vi "Day 24-With Map.vi"() -> ()   [LabVIEW 2021]
uses:
  Day 24-Operation Enum.ctl
  Day 24-Variable Enum.ctl
  <vilib>/Utility/file.llb/Read Delimited Spreadsheet (string).vi
panel:
  out "Array 2":T3(array[cluster])
  out "Model Number":u64
  out "Array":T4(array[cluster])
  in  "Input File":enum32{"example input", "input"}(radio)
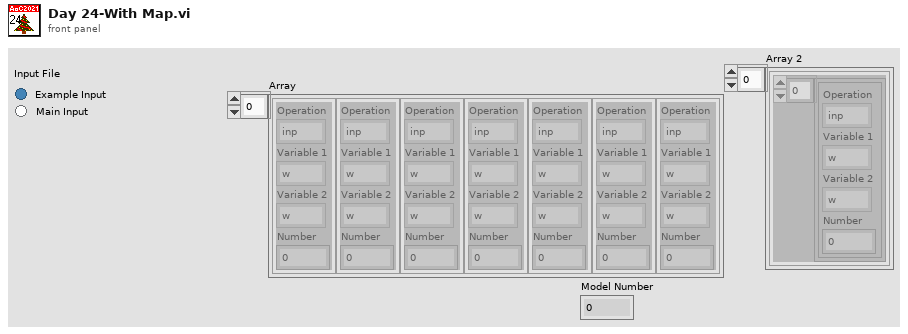
[diagram p1: front panel]
types:
  T1 = typedef "Day 24-Operation Enum.ctl" = enum16{"inp", "add", "mul", "div", "mod", "eql"}
  T2 = typedef "Day 24-Variable Enum.ctl" = enum16{"w", "x", "y", "z", "num"}
  T3 = cluster{cluster{"Operation":T1, "Variable 1":T2, "Variable 2":T2, "Number":i64}[]}[]
  T4 = cluster{"Operation":T1, "Variable 1":T2, "Variable 2":T2, "Number":i64}[]
  T5 = cluster{"Operation":T1, "Variable 1":T2, "Variable 2":T2, "Number":i64}
  T6 = cluster{cluster{"Operation":T1, "Variable 1":T2, "Variable 2":T2, "Number":i64}[]}
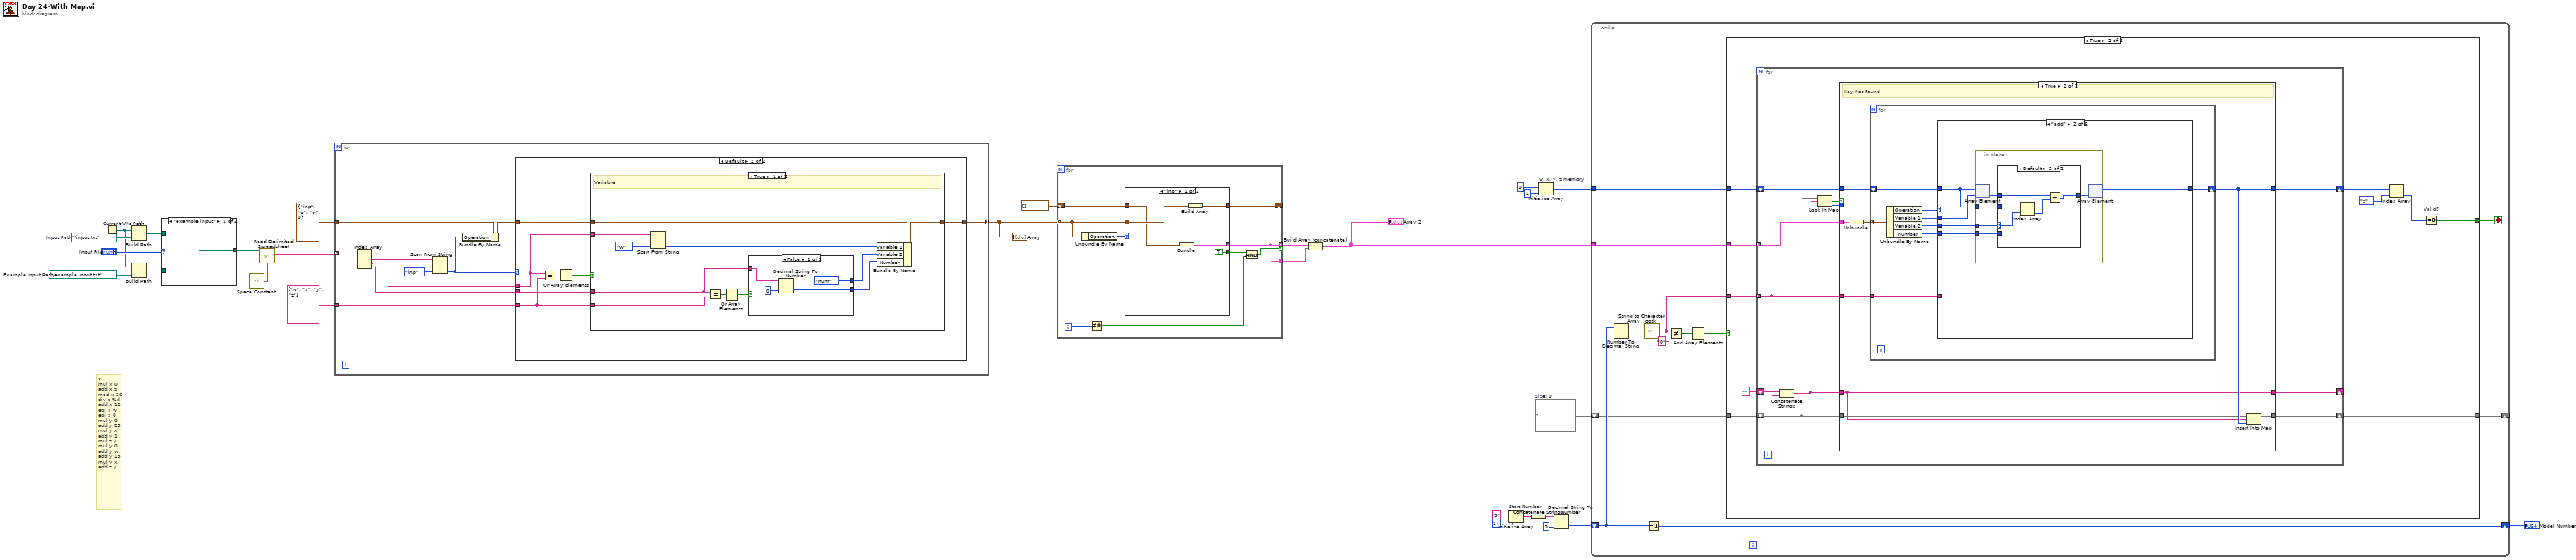
[diagram p0: block diagram]
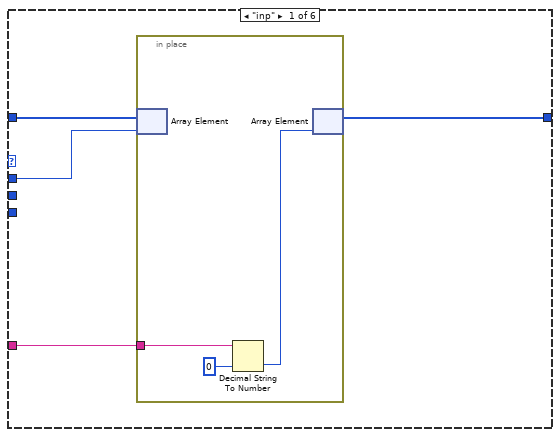
[diagram p4: hidden frame]
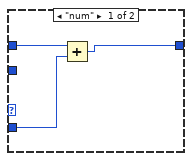
[diagram p5: hidden frame]
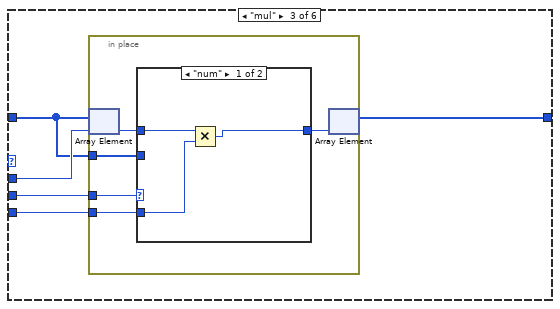
[diagram p6: hidden frame]
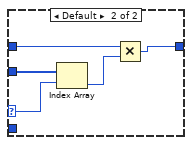
[diagram p7: hidden frame]
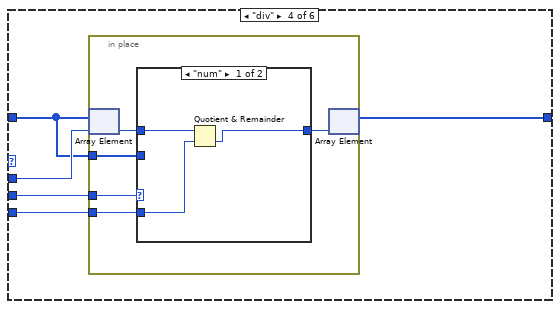
[diagram p8: hidden frame]
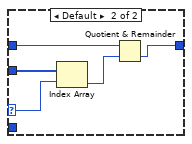
[diagram p9: hidden frame]
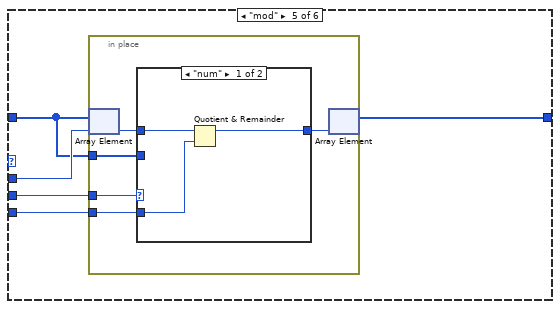
[diagram p10: hidden frame]
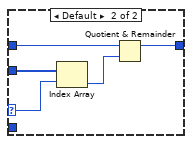
[diagram p11: hidden frame]
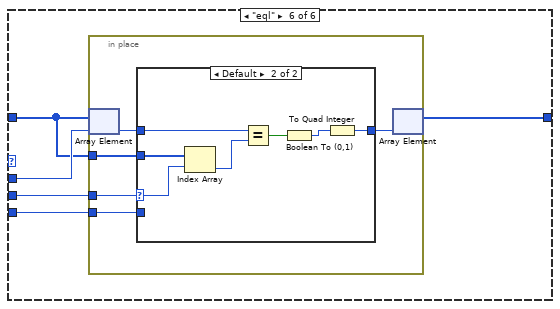
[diagram p12: hidden frame]
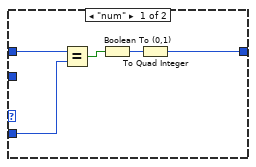
[diagram p13: hidden frame]
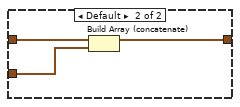
[diagram p14: hidden frame]
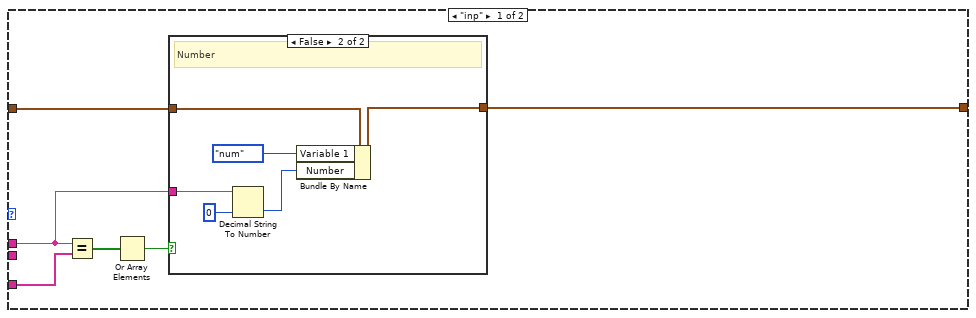
[diagram p15: hidden frame]
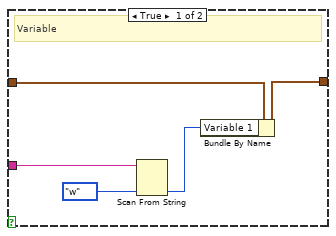
[diagram p16: hidden frame]
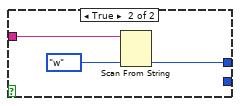
[diagram p17: hidden frame]
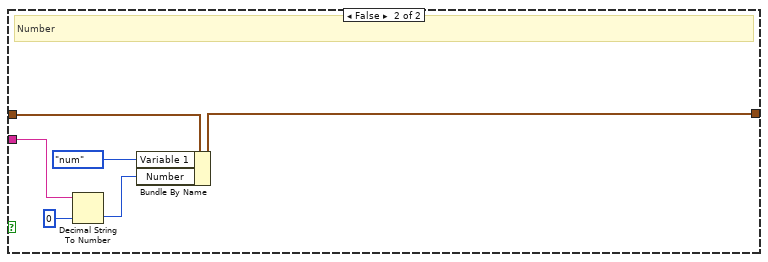
[diagram p18: hidden frame]
diagram:
  w4 = map{string, i64[]} {}  # Size: 0
  w26 = path "../example input.txt"  # Example Input Path
  w27 = path "../input.txt"  # Input Path
  # "w\nmul x 0\nadd x z\nmod x 26\ndiv z %d\nadd x 12\neql x w\neql x 0\nmul y 0\nadd y 25\nmul y x\nadd y 1\nmul z y\nmul y 0\nadd y w\nadd y 15\nmul y x\nadd z y"
  n1 = Current VI's Path() -> (path=w22:path)
  n2 = Build Path(base path=w22, name or relative path=w27) -> (appended path=w24:path)
  n3 = Build Path(base path=w22, name or relative path=w26) -> (appended path=w23:path)
  n4 = case shown="\"example input\"" "Input File" {
    tunnel: w24 -> [_ w29]
    tunnel: w23 -> [w28 _]
    tunnel: [w28 w29] -> w1
    frame "example input" {
    }
    frame "input" {
    }
  }
  n5 = call <vilib>:"Space Constant.vi"() -> ("String"=w19:string)
  n6 = call-poly <vilib>:"Read Delimited Spreadsheet.vi"("file path (dialog if empty)"=w1, "delimiter (\\t)"=w19) -> ("all rows"=w18:string[][])  [unwired: 8 in, 5 out]
  n7 = for {
    tunnel: w18 -> [w34] mode=indexing
    tunnel: string[] ["w", "x", "y", "z"] -> [w39]
    tunnel: T5 {"Operation"=enum."inp", "Variable 1"=enum."w", "Variable 2"=enum."w", "Number"=0} -> [w37]
    tunnel: [w35] -> w17 mode=indexing
    n8 = Index Array(array=w34) -> (element #1=w33:string, element #2=w31:string, element #3=w30:string)  [unwired: 3 in]
    n9 = Scan From String(input string=w33, default 1=Day_24-Operation_Enum."inp") -> (output 1=w36:T1)  [unwired: 3 in, 3 out]
    n10 = Bundle By Name(cluster=w37, "Operation"=w36) -> (w38:T5)
    n11 = case shown="Default" w36 {
      tunnel: w39 -> [w45 w59]
      tunnel: w38 -> [w42 w61]
      tunnel: [w41 w60] -> w35
      tunnel: w31 -> [w40 w58]
      tunnel: w30 -> [_ w57]
      frame "inp" {
        n12 = Equal?(x=w40, y=w45) -> (x = y?=w44:bool[])
        n13 = Or Array Elements(Boolean array=w44) -> (logical OR=w43:bool)
        n14 = case shown="False" w43 {
          tunnel: w42 -> [w50 w56]
          tunnel: w40 -> [w49 w54]
          tunnel: [w46 w55] -> w41
          frame True {
            # "Variable"
            n15 = Scan From String(input string=w49, default 1=Day_24-Variable_Enum."w" ("Variable 1")) -> (output 1=w47:T2)  [unwired: 3 in, 3 out]
            n16 = Bundle By Name(cluster=w50, "Variable 1"=w47) -> (w46:T5)
          }
          frame False {
            # "Number"
            n17 = Decimal String To Number(string=w54, default (0L)=i64 0 ("default (0 I32)")) -> (number=w52:i64)  [unwired: 1 in, 1 out]
            n18 = Bundle By Name(cluster=w56, "Variable 1"=Day_24-Variable_Enum."num", "Number"=w52) -> (w55:T5)
          }
        }
      }
      frame Default {
        n19 = Equal?(x=w58, y=w59) -> (x = y?=w63:bool[])
        n20 = Or Array Elements(Boolean array=w63) -> (logical OR=w62:bool)
        n21 = case shown="True" w62 {
          tunnel: w61 -> [w74 w87]
          tunnel: w58 -> [w73 w85]
          tunnel: [w70 w86] -> w60
          tunnel: w59 -> [w68 _]
          tunnel: w57 -> [w64 _]
          frame True {
            # "Variable"
            n22 = Scan From String(input string=w73, default 1=Day_24-Variable_Enum."w" ("Variable 1")) -> (output 1=w71:T2)  [unwired: 3 in, 3 out]
            n23 = Equal?(x=w64, y=w68) -> (x = y?=w69:bool[])
            n24 = Or Array Elements(Boolean array=w69) -> (logical OR=w67:bool)
            n25 = case shown="False" w67 {
              tunnel: w64 -> [w78 w80]
              tunnel: [Day_24-Variable_Enum."num" ("Variable 1") w79] -> w66
              tunnel: [w77 _] -> w65
              frame False {
                n26 = Decimal String To Number(string=w78, default (0L)=i64 0 ("default (0 I32)")) -> (number=w77:i64)  [unwired: 1 in, 1 out]
              }
              frame True {
                n27 = Scan From String(input string=w80, default 1=Day_24-Variable_Enum."w" ("Variable 1")) -> (output 1=w79:T2)  [unwired: 3 in, 3 out]
              }
            }
            n28 = Bundle By Name(cluster=w74, "Variable 1"=w71, "Variable 2"=w66, "Number"=w65) -> (w70:T5)
          }
          frame False {
            # "Number"
            n29 = Decimal String To Number(string=w85, default (0L)=i64 0 ("default (0 I32)")) -> (number=w83:i64)  [unwired: 1 in, 1 out]
            n30 = Bundle By Name(cluster=w87, "Variable 1"=Day_24-Variable_Enum."num", "Number"=w83) -> (w86:T5)
          }
        }
      }
    }
  }
  "Array" <- w17
  n31 = for {
    tunnel: w17 -> [w95] mode=indexing
    shift-right: [w94] -> _
    shift-left: T4 [] -> [w93]
    tunnel: [w88] -> w5 mode=indexing if=w91
    tunnel: [w88] -> w2
    i -> [w90]
    n32 = Unbundle By Name(w95) -> ("Operation"=w96:T1)
    n33 = Not Equal To 0?(x=w90) -> (x != 0?=w89:bool)
    n34 = case shown="\"inp\"" w96 {
      tunnel: w95 -> [w101 w104]
      tunnel: [w100 w103] -> w94
      tunnel: w93 -> [w98 w102]
      tunnel: [w99 _] -> w88
      tunnel: [TRUE _] -> w92
      frame "inp" {
        n35 = Bundle(w98) -> (w99:T6)  [unwired: 1 in]
        n36 = Build Array(w101) -> (w100:T4)
      }
      frame Default {
        n37 = Build Array (concatenate)(w102, w104) -> (w103:T4)
      }
    }
    n38 = And(x=w92, y=w89) -> (x .and. y?=w91:bool)
  }
  n39 = Build Array (concatenate)(w5, w2) -> (w3:T3)
  "Array 2" <- w3
  n40 = Initialize Array "Start Number"("9", 14 ("dimension size")) -> (w10:string[])
  n41 = Concatenate Strings(w10) -> (w9:string)
  n42 = Initialize Array "w, x, y, z memory"(i64 0, 4 ("dimension size")) -> (w13:i64[])
  n43 = Decimal String To Number(string=w9, default (0L)=u64 0 ("default (0 I32)")) -> (number=w7:u64)  [unwired: 1 in, 1 out]
  n44 = while {
    tunnel: w13 -> [w116]
    shift-right: [w108] -> w6
    shift-left: w7 -> [w110]
    tunnel: w3 -> [w107]
    shift-right: [w106] -> _
    shift-left: w4 -> [w105]
    stop <- w115 stop-if-true
    n45 = Number To Decimal String(number=w110) -> (decimal integer string=w113:string)  [unwired: 1 in]
    n46 = call <userlib>:"String to Character Array__ogtk.vi"("Input String"=w113) -> ("Character Array"=w111:string[])
    n47 = Decrement(x=w110) -> (x-1=w108:u64)
    n48 = Not Equal?(x=w111, y="0") -> (x != y?=w112:bool[])
    n49 = And Array Elements(Boolean array=w112) -> (logical AND=w109:bool)
    n50 = case shown="True" w109 {
      tunnel: w116 -> [_ w127]
      tunnel: [_ w124] -> w115
      tunnel: w111 -> [_ w123]
      tunnel: w107 -> [_ w121]
      tunnel: [w117 w119] -> w106
      tunnel: w105 -> [w117 w118]
      frame False {
      }
      frame True {
        n51 = for {
          shift-right: [w136] -> w126
          shift-left: w127 -> [w138]
          tunnel: w123 -> [w132] mode=indexing
          tunnel: w121 -> [w137] mode=indexing
          shift-right: [w128] -> _
          shift-left: "" -> [w133]
          shift-right: [w129] -> w119
          shift-left: w118 -> [w130]
          n52 = Concatenate Strings(w133, w132) -> (w131:string)
          n53 = Look In Map(map=w130, key=w131) -> (key not found?=w135:bool, value=w134:i64[])  [unwired: 1 in]
          n54 = case shown="True" w135 {
            tunnel: w138 -> [_ w149]
            tunnel: w137 -> [_ w148]
            tunnel: w132 -> [_ w146]
            tunnel: [w141 w145] -> w136
            tunnel: w134 -> [w141 _]
            tunnel: w131 -> [w140 w142]
            tunnel: w130 -> [w139 w144]
            tunnel: [w139 w143] -> w129
            tunnel: [w140 w142] -> w128
            frame False {
              # "Key Found"
            }
            frame True {
              # "Key Not Found"
              n55 = Unbundle(w148) -> (w147:T4)
              n56 = for {
                tunnel: w147 -> [w157] mode=indexing
                tunnel: w146 -> [w150]
                shift-right: [w153] -> w145
                shift-left: w149 -> [w155]
                n57 = Unbundle By Name(w157) -> ("Operation"=w156:T1, "Variable 1"=w154:T2, "Variable 2"=w152:T2, "Number"=w151:i64)
                n58 = case shown="\"add\"" w156 {
                  tunnel: w155 -> [w161 w167 w185 w203 w221 w239]
                  tunnel: w154 -> [w160 w169 w187 w205 w223 w241]
                  tunnel: [w159 w168 w186 w204 w222 w240] -> w153
                  tunnel: w152 -> [_ w166 w184 w202 w220 w238]
                  tunnel: w151 -> [_ w165 w183 w201 w219 w237]
                  tunnel: w150 -> [w158 _ _ _ _ _]
                  frame "inp" {
                    n59 = in-place {
                      in-place-border: w158 -> [w162]
                      n60 = in-place-array #1(w161, w160) -> ()  [unwired: 1 out]
                      n61 = Decimal String To Number(string=w162, default (0L)=i64 0 ("default (0 I32)")) -> (number=w163:i64)  [unwired: 1 in, 1 out]
                      n62 = in-place-array #1(w163) -> (w159:i64[])  [unwired: 1 out]
                    }
                  }
                  frame "add" {
                    n63 = in-place {
                      in-place-border: w167 -> [w172]
                      in-place-border: w166 -> [w174]
                      in-place-border: w165 -> [w170]
                      n64 = in-place-array #2(w167, w169) -> (w173:i64)
                      n65 = case shown="Default" w174 {
                        selector: w174 -> [_ w181]
                        tunnel: w173 -> [w177 w180]
                        tunnel: w172 -> [_ w182]
                        tunnel: [w175 w178] -> w171
                        tunnel: w170 -> [w176 _]
                        frame "num" {
                          n66 = Add(x=w177, y=w176) -> (x+y=w175:i64)
                        }
                        frame Default {
                          n67 = Index Array(array=w182, index=w181) -> (element=w179:i64)
                          n68 = Add(x=w180, y=w179) -> (x+y=w178:i64)
                        }
                      }
                      n69 = in-place-array #2(w171) -> (w168:i64[])  [unwired: 1 out]
                    }
                  }
                  frame "mul" {
                    n70 = in-place {
                      in-place-border: w185 -> [w190]
                      in-place-border: w184 -> [w192]
                      in-place-border: w183 -> [w188]
                      n71 = in-place-array #3(w185, w187) -> (w191:i64)
                      n72 = case shown="\"num\"" w192 {
                        selector: w192 -> [_ w199]
                        tunnel: w191 -> [w195 w198]
                        tunnel: w190 -> [_ w200]
                        tunnel: [w193 w196] -> w189
                        tunnel: w188 -> [w194 _]
                        frame "num" {
                          n73 = Multiply(x=w195, y=w194) -> (x*y=w193:i64)
                        }
                        frame Default {
                          n74 = Index Array(array=w200, index=w199) -> (element=w197:i64)
                          n75 = Multiply(x=w198, y=w197) -> (x*y=w196:i64)
                        }
                      }
                      n76 = in-place-array #3(w189) -> (w186:i64[])  [unwired: 1 out]
                    }
                  }
                  frame "div" {
                    n77 = in-place {
                      in-place-border: w203 -> [w208]
                      in-place-border: w202 -> [w210]
                      in-place-border: w201 -> [w206]
                      n78 = in-place-array #4(w203, w205) -> (w209:i64)
                      n79 = case shown="\"num\"" w210 {
                        selector: w210 -> [_ w217]
                        tunnel: w209 -> [w213 w216]
                        tunnel: w208 -> [_ w218]
                        tunnel: [w211 w214] -> w207
                        tunnel: w206 -> [w212 _]
                        frame "num" {
                          n80 = Quotient & Remainder(x=w213, y=w212) -> (floor(x/y)=w211:i64)  [unwired: 1 out]
                        }
                        frame Default {
                          n81 = Index Array(array=w218, index=w217) -> (element=w215:i64)
                          n82 = Quotient & Remainder(x=w216, y=w215) -> (floor(x/y)=w214:i64)  [unwired: 1 out]
                        }
                      }
                      n83 = in-place-array #4(w207) -> (w204:i64[])  [unwired: 1 out]
                    }
                  }
                  frame "mod" {
                    n84 = in-place {
                      in-place-border: w221 -> [w226]
                      in-place-border: w220 -> [w228]
                      in-place-border: w219 -> [w224]
                      n85 = in-place-array #5(w221, w223) -> (w227:i64)
                      n86 = case shown="\"num\"" w228 {
                        selector: w228 -> [_ w235]
                        tunnel: w227 -> [w231 w234]
                        tunnel: w226 -> [_ w236]
                        tunnel: [w229 w232] -> w225
                        tunnel: w224 -> [w230 _]
                        frame "num" {
                          n87 = Quotient & Remainder(x=w231, y=w230) -> (x-y*floor(x/y)=w229:i64)  [unwired: 1 out]
                        }
                        frame Default {
                          n88 = Index Array(array=w236, index=w235) -> (element=w233:i64)
                          n89 = Quotient & Remainder(x=w234, y=w233) -> (x-y*floor(x/y)=w232:i64)  [unwired: 1 out]
                        }
                      }
                      n90 = in-place-array #5(w225) -> (w222:i64[])  [unwired: 1 out]
                    }
                  }
                  frame "eql" {
                    n91 = in-place {
                      in-place-border: w239 -> [w244]
                      in-place-border: w238 -> [w246]
                      in-place-border: w237 -> [w242]
                      n92 = in-place-array #6(w239, w241) -> (w245:i64)
                      n93 = case shown="Default" w246 {
                        selector: w246 -> [_ w257]
                        tunnel: w245 -> [w251 w256]
                        tunnel: w244 -> [_ w258]
                        tunnel: [w247 w252] -> w243
                        tunnel: w242 -> [w250 _]
                        frame "num" {
                          n94 = Equal?(x=w251, y=w250) -> (x = y?=w249:bool)
                          n95 = Boolean To (0,1)(Boolean=w249) -> (0, 1=w248:i16)
                          n96 = To Quad Integer(1:w248) -> (0:w247:i64)
                        }
                        frame Default {
                          n97 = Index Array(array=w258, index=w257) -> (element=w255:i64)
                          n98 = Equal?(x=w256, y=w255) -> (x = y?=w254:bool)
                          n99 = Boolean To (0,1)(Boolean=w254) -> (0, 1=w253:i16)
                          n100 = To Quad Integer(1:w253) -> (0:w252:i64)
                        }
                      }
                      n101 = in-place-array #6(w243) -> (w240:i64[])  [unwired: 1 out]
                    }
                  }
                }
              }
              n102 = Insert Into Map(map in=w144, key=w142, value=w145) -> (map out=w143:map{string, i64[]})  [unwired: 2 out]
            }
          }
        }
        n103 = Index Array(array=w126, index=Day_24-Variable_Enum."z" ("Variable 1")) -> (element=w122:i64)
        n104 = Equal To 0? "Valid?"(x=w122) -> (x = 0?=w124:bool)
      }
    }
  }
  "Model Number" <- w6
